vi "test_pcap.vi"() -> ()   [LabVIEW 2020]
uses:
  libpcaplv/libpcaplv.lvlib
panel:
  in  "payload":u8[](array[numeric])=[3, 0, 0, 0, 0, 60, 2, 0, 0, 1, 33, 32, 8, 0, 69, 0, 0, 128, 0, 0, 64, 0, 1, 17, 109, 79, 10, 1, 33, 1, 224, 224, 0, 60, 0, 1, 0, 1, 0, 108, 0, 0, 207, 99, 155, 15, 106, 80, 222, 38, 87, 135, 73, 82, 67, 38, 174, 247, 142, 66, 65, 133, 227, 190, 153, 102, 234, 106, 114, 88, 44, 57, 78, 20, 118, 109, 162, 179, 100, 58, 251, 232, 27, 218, 230, 200, 194, 136, 100, 49, 35, 190, 183, 206, 140, 143, 59, 50, 170, 143, 191, 177, 50, 202, 166, 88, 17, 70, 246, 221, 189, 91, 198, 95, 193, 99, 124, 227, 186, 214, 255, 207, 114, 246, 55, 242, 29, 9, 249, 8, 63, 31, 139, 229, 65, 28, 152, 166, 57, 36, 219, 238, 0, 40, 227, 49, 212, 0] format="%.0x"
  in  "# of payloads":i32=1
  in  "interval uS":i32=10000
  in  "capture file path":path=path "../testWin.pcap"
  out "error out":errorcluster
  in  "timeval":cluster{"time_t":u64, "useconds_t":u64}
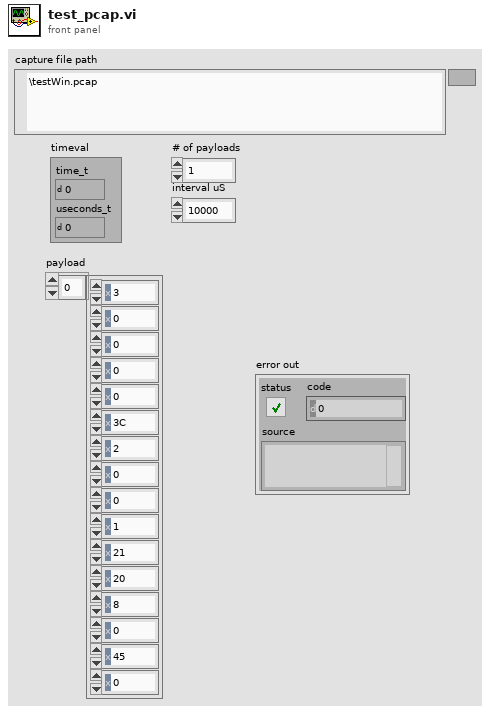
[diagram p1: front panel]
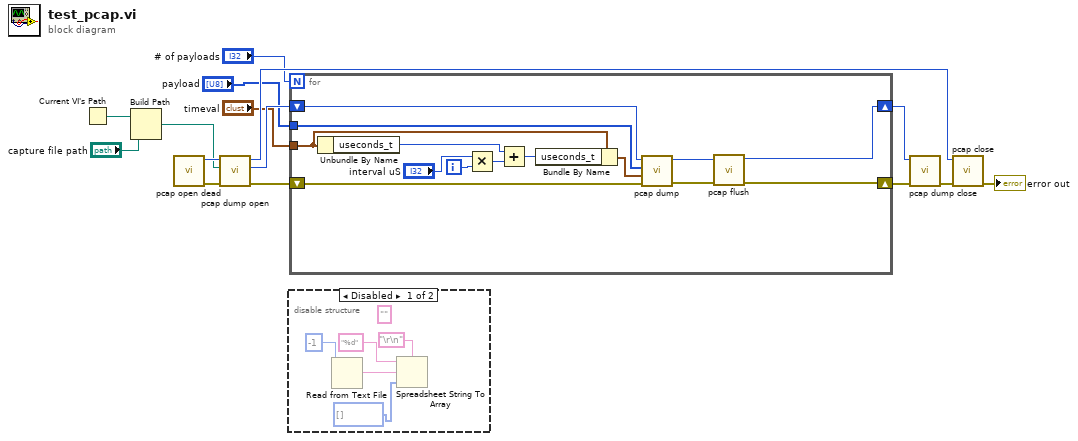
[diagram p0: block diagram]
diagram:
  n1 = Current VI's Path() -> (path=w3:path)
  n2 = Build Path(base path=w3, name or relative path="capture file path") -> (appended path=w1:path)
  n3 = call "pcap open dead.vi"() -> ("error out"=w12:errorcluster, "pcap_t"=w11:u64)  [unwired: 10 in]
  n4 = call "pcap dump open.vi"("error in"=w12, "capture file path"=w1, "pcap_t in"=w11) -> ("error out"=w7:errorcluster, "pcap_dumper_t"=w15:u64, "pcap_t out"=w9:u64)  [unwired: 6 in]
  n5 = disable-structure shown="Disabled" {
    frame Disabled {
      (unwired) ""
      n6 = Read from Text File(count=-1) -> (text=w19:string)  [unwired: 3 in, 3 out]
      n7 = Spreadsheet String To Array(delimiter (Tab)="\r\n", format string="%d", spreadsheet string=w19, array type (2D Dbl)=u8[] []) -> ()  [unwired: 1 out]
    }
    frame Enabled {
    }
  }
  n8 = for {
    N: "# of payloads" -> [_]
    shift-right: [w21] -> w14
    shift-left: w15 -> [w34]
    shift-right: [w22] -> w13
    shift-left: w7 -> [w33]
    tunnel: "timeval" -> [w28]
    tunnel: "payload" -> [w25]
    i -> [w32]
    n9 = Unbundle By Name(w28) -> ("useconds_t"=w31:u64)
    n10 = Multiply(x="interval uS", y=w32) -> (x*y=w30:i32)
    n11 = Add(x=w31, y=w30) -> (x+y=w27:u64)
    n12 = Bundle By Name(cluster=w28, "useconds_t"=w27) -> (w26:cluster{"time_t":u64, "useconds_t":u64})
    n13 = call "pcap dump.vi"("error in"=w33, "timeval"=w26, "Packet in"=w25, "pcap_dumper_t in"=w34) -> ("error out"=w23:errorcluster, "pcap_dumper_t out"=w24:u64)  [unwired: 6 in]
    n14 = call "pcap flush.vi"("error in"=w23, "pcap_dumper_t in"=w24) -> ("error out"=w22:errorcluster, "pcap_dumper_t out"=w21:u64)  [unwired: 8 in]
  }
  n15 = call "pcap dump close.vi"("error in"=w13, "pcap_dumper_t in"=w14) -> ("error out"=w10:errorcluster)  [unwired: 9 in]
  n16 = call "pcap close.vi"("error in"=w10, "pcap_t in"=w9) -> ("error out"=→"error out":errorcluster)  [unwired: 9 in]
